vi "Boolean 2D Array to Int Array.vi"(5 "Mode":enum16{"to Array", "to Number"}(ring), 7 "Array of Boolean":bool[][](array[boolean])) -> (0 "Array out":u32[][](array[numeric]))   [LabVIEW 2014]
doc: "<B>Copyright</B>: (c) MHWirth 2015. All rights reserved.\n\nThis subVI recieves an 1D array of Boolean and converts this to a number or an array of (0,1).\n\n<B>to Number</B>: The boolean array is converted to one number (U32). To retreive the boolean array, you should use <B>Number to Boolean Array<\\B> function.\n\n<B>to Array</B>: The boolean aray is converted to array of (0,1) (array of U32)."
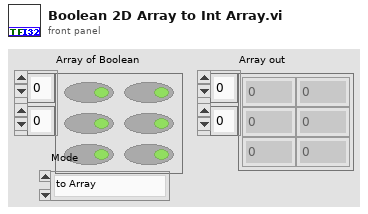
[diagram p1: front panel]
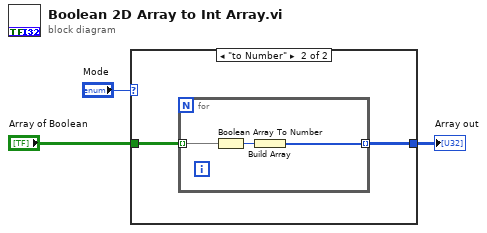
[diagram p0: block diagram]
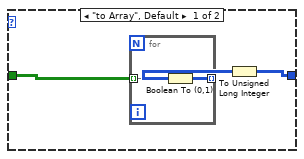
[diagram p2: hidden frame]
diagram:
  n1 = case shown="\"to Number\"" "Mode" {
    tunnel: "Array of Boolean" -> [w6 w10]
    tunnel: [w4 w9] -> w1
    frame "to Array", Default {
      n2 = for {
        tunnel: w6 -> [w8] mode=indexing
        tunnel: [w7] -> w5 mode=indexing
        n3 = Boolean To (0,1)(Boolean=w8) -> (0, 1=w7:i16[])
      }
      n4 = To Unsigned Long Integer(number=w5) -> (unsigned 32bit integer=w4:u32[][])
    }
    frame "to Number" {
      n5 = for {
        tunnel: w10 -> [w11] mode=indexing
        tunnel: [w12] -> w9 mode=indexing
        n6 = Boolean Array To Number(Boolean array=w11) -> (number=w13:u32)
        n7 = Build Array(w13) -> (w12:u32[])
      }
    }
  }
  "Array out" <- w1
